vi "Get Local XML Path.vi"(8 "Error In":errorcluster) -> (0 "Error Out":errorcluster, 2 "Found ?":bool, 3 "XML Path":path)   [LabVIEW 2019, in "Project XML Editor.lvclass"]
uses:
  Project XML Editor.lvclass
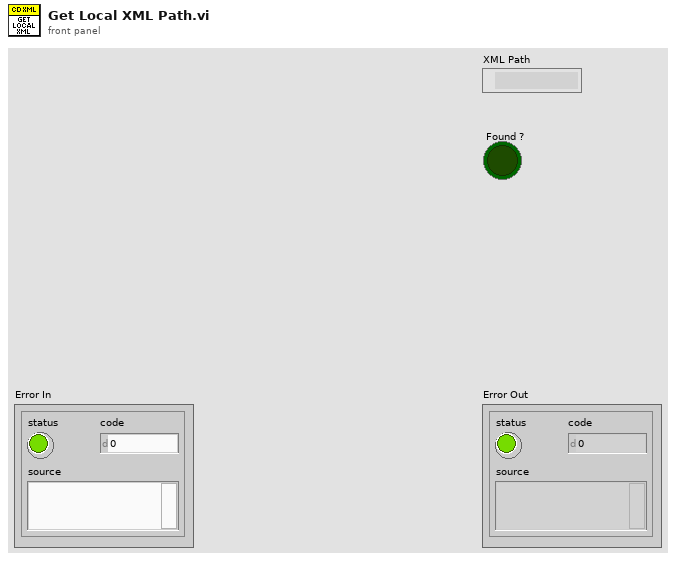
[diagram p1: front panel]
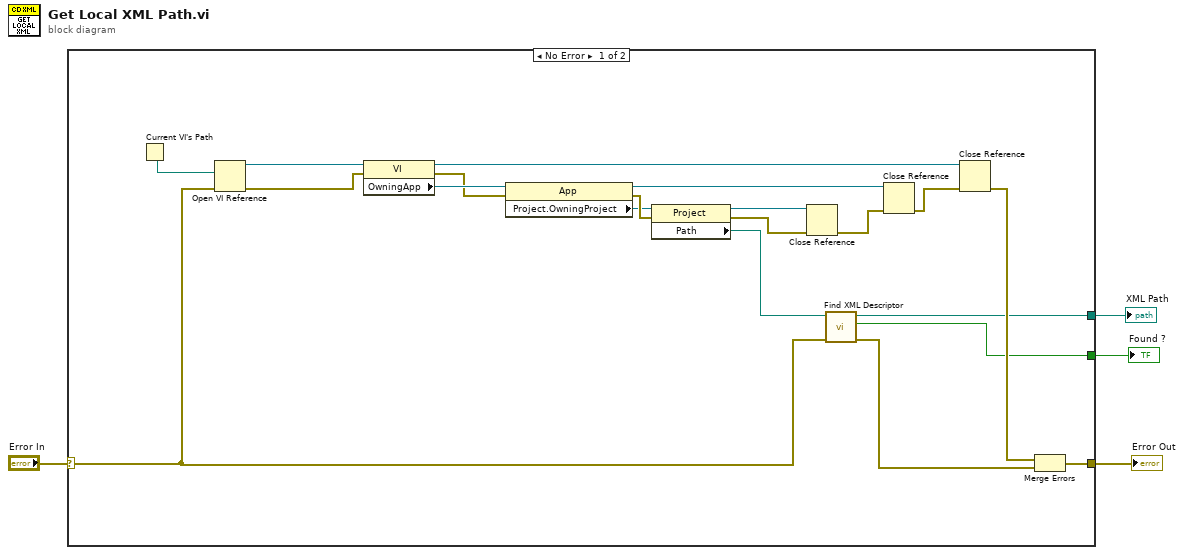
[diagram p0: block diagram]
diagram:
  n1 = case shown="No Error" "Error In" {
    selector: "Error In" -> [w10 w25]
    tunnel: [w7 w25] -> w3
    tunnel: [w6 _] -> w2
    tunnel: [w5 _] -> w1
    frame No Error {
      n2 = Current VI's Path() -> (path=w22:path)
      n3 = Open VI Reference(vi path=w22, error in (no error)=w10) -> (vi reference=w21:refnum<vi>, error out=w20:errorcluster)  [unwired: 4 in]
      n4 = property class="VI"(reference=w21, error in=w20) -> (reference out=w17:refnum<vi>, error out=w18:errorcluster, "OwningApp"=w19:refnum<vi>)
      n5 = property class="App"(reference=w19, error in=w18) -> (reference out=w16:refnum<vi>, error out=w24:errorcluster, "Project.OwningProject"=w23:refnum<vi>)
      n6 = property class="Project"(reference=w23, error in=w24) -> (reference out=w15:refnum<vi>, error out=w14:errorcluster, "Path"=w11:path)
      n7 = Close Reference(reference=w15, error in (no error)=w14) -> (error out=w13:errorcluster)
      n8 = call "Find XML Descriptor.vi"("error in"=w10, "Project Path"=w11) -> ("error out"=w9:errorcluster, "Found ?"=w5:bool, "XML Path"=w6:path)  [unwired: 7 in]
      n9 = Close Reference(reference=w16, error in (no error)=w13) -> (error out=w12:errorcluster)
      n10 = Close Reference(reference=w17, error in (no error)=w12) -> (error out=w8:errorcluster)
      n11 = Merge Errors(w8, w9) -> (w7:errorcluster)
    }
    frame Error {
    }
  }
  "Error Out" <- w3
  "XML Path" <- w2
  "Found ?" <- w1
